vi "Dispatch Verify Queue.vi"(8 "error in (no error)":errorcluster, 9 "Timeout (100 ms)":i32=100, 10 "queue name":string, 11 "receiver host":string) -> (0 "error out":errorcluster, 2 "String Response":string, 3 "Message":T1)   [LabVIEW 2014, in "AMC.lvlib"]
uses:
  AMC.lvlib
  _SubVIs/Globals.vi
  Keyed Array/KeyedArray.ctl
  Keyed Array/Tools_KeyedArray.lvlib
  _SubVIs/TypeDefs/Message.ctl
panel:
  out "Response time (ms)":i32
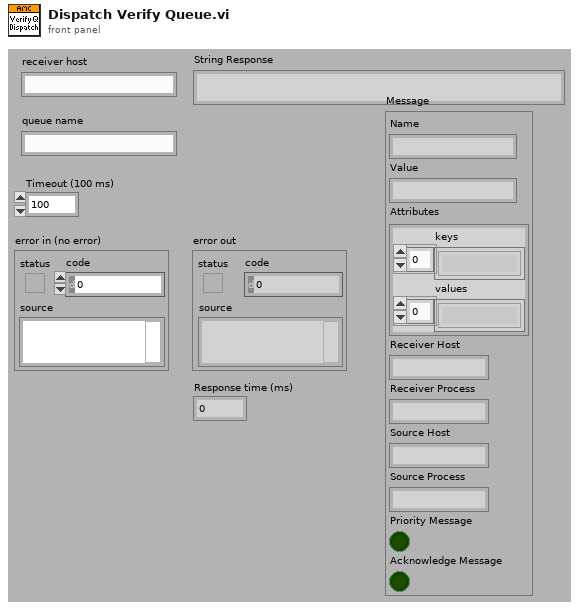
[diagram p1: front panel]
types:
  T1 = typedef "AMC.lvlib/Message.ctl" = cluster{"Name":string, "Value":string, "Attributes":T2, "Receiver Host":string, "Receiver Process":string, "Source Host":string, "Source Process":string, "Priority Message":bool, "Acknowledge Message":bool}
  T2 = typedef "Tools_KeyedArray.lvlib/KeyedArray.ctl" = cluster{"keys":string[], "values":string[]}
  T3 = typedef "AMC.lvlib/Message Queue.ctl" = refnum<queue>
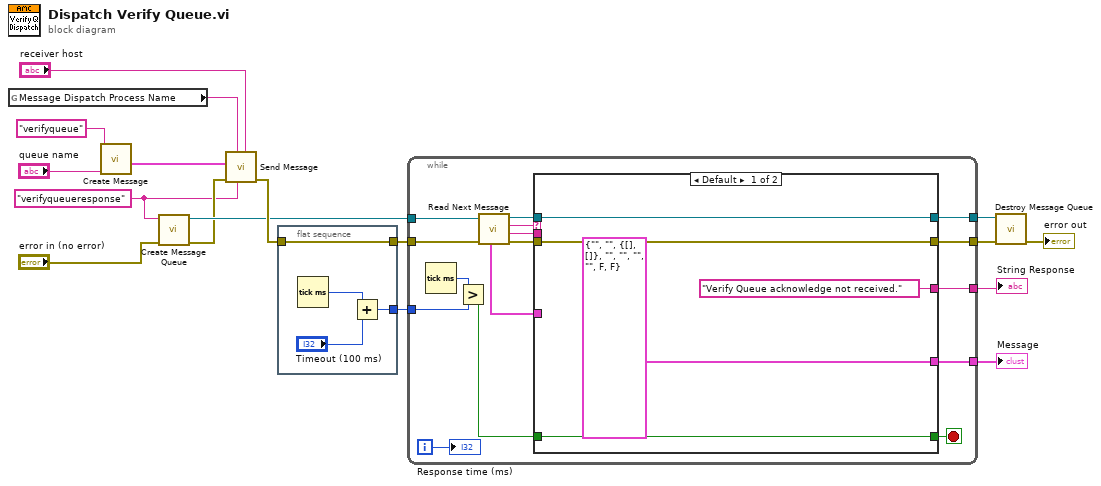
[diagram p0: block diagram]
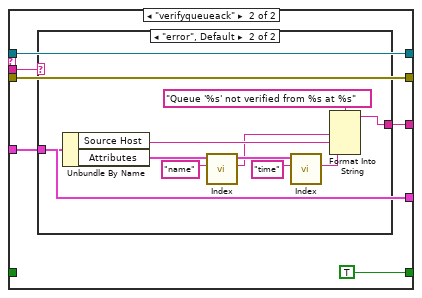
[diagram p2: hidden frame]
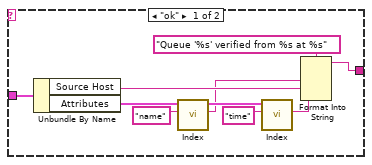
[diagram p3: hidden frame]
diagram:
  w3 = "verifyqueueresponse" ("message queue name")
  n1 = global read "Globals.vi" "Message Dispatch Process Name"() -> (w1:string)
  n2 = call "Create Message.vi"("Value"="queue name", "Name"="verifyqueue") -> ("Message"=w4:T1)  [unwired: 1 in, 8 out]
  n3 = call "Create Message Queue.vi"("error in (no error)"="error in (no error)", "Message Queue Name"=w3) -> ("error out"=w5:errorcluster, "Message Queue out"=w6:T3)  [unwired: 2 in, 6 out]
  n4 = call "Send Message.vi"("Receiver Host"="receiver host", "Source Process"=w3, "Receiver Process"=w1, "error in (no error)"=w5, "Message"=w4) -> ("error out"=w11:errorcluster)  [unwired: 3 in, 3 out]
  n5 = flat-sequence {
    tunnel: [w21] -> w10
    tunnel: w11 -> [w21]
    tunnel: [w18] -> w9
    frame #0 {
      n6 = Tick Count (ms)() -> (millisecond timer value=w20:u32)
      n7 = Add(x=w20, y="Timeout (100 ms)") -> (x+y=w18:u32)
    }
  }
  n8 = while {
    tunnel: w10 -> [w37]
    tunnel: [w34] -> w14
    tunnel: [w33] -> w13
    tunnel: [w30] -> w7
    tunnel: [w29] -> w8
    tunnel: w6 -> [w28]
    tunnel: w9 -> [w26]
    i -> [w23]
    stop <- w25 stop-if-true
    n9 = Tick Count (ms)() -> (millisecond timer value=w27:u32)
    n10 = Greater?(x=w27, y=w26) -> (0:w24:bool)
    n11 = call "Read Next Message.vi"("error in (no error)"=w37, "Message Queue in"=w28) -> ("error out"=w32:errorcluster, "Message Value"=w22:string, "Message Name"=w36:string, "Message Queue out"=w31:T3, "Message"=w35:T1)  [unwired: 3 in, 2 out]
    n12 = case shown="Default" w36 {
      tunnel: w35 -> [_ w47]
      tunnel: ["Verify Queue acknowledge not received." w48] -> w34
      tunnel: [T1 {"Name"="", "Value"="", "Attributes"={"keys"=[], "values"=[]}, "Receiver Host"="", "Receiver Process"="", "Source Host"="", "Source Process"="", "Priority Message"=FALSE, "Acknowledge Message"=FALSE} ("Message") w47] -> w33
      tunnel: [w39 w46] -> w30
      tunnel: w32 -> [w39 w46]
      tunnel: [w40 w45] -> w29
      tunnel: w31 -> [w40 w45]
      tunnel: [w38 TRUE] -> w25
      tunnel: w24 -> [w38 _]
      tunnel: w22 -> [_ w43]
      frame Default {
      }
      frame "verifyqueueack" {
        n13 = case shown="\"error\", Default" w43 {
          tunnel: [w54 w64] -> w48
          tunnel: w47 -> [w53 w63]
          frame "ok" {
            n14 = Unbundle By Name(w53) -> ("Source Host"=w58:string, "Attributes"=w51:T2)
            n15 = call "Index.vi"("key"="name", "array in"=w51) -> ("value"=w49:string, "duplicate array"=w50:T2)  [unwired: 2 in, 2 out]
            n16 = call "Index.vi"("key"="time", "array in"=w50) -> ("value"=w57:string)  [unwired: 2 in, 3 out]
            n17 = Format Into String(format string="Queue '%s' verified from %s at %s", w49, w58, w57) -> (resulting string=w54:string)  [unwired: 2 in, 1 out]
          }
          frame "error", Default {
            n18 = Unbundle By Name(w63) -> ("Source Host"=w68:string, "Attributes"=w61:T2)
            n19 = call "Index.vi"("key"="name", "array in"=w61) -> ("value"=w59:string, "duplicate array"=w60:T2)  [unwired: 2 in, 2 out]
            n20 = call "Index.vi"("key"="time", "array in"=w60) -> ("value"=w67:string)  [unwired: 2 in, 3 out]
            n21 = Format Into String(format string="Queue '%s' not verified from %s at %s", w59, w68, w67) -> (resulting string=w64:string)  [unwired: 2 in, 1 out]
          }
        }
      }
    }
    "Response time (ms)" <- w23
  }
  "String Response" <- w14
  "Message" <- w13
  n22 = call "Destroy Message Queue.vi"("error in (no error)"=w7, "Message Queue in"=w8) -> ("error out"=→"error out":errorcluster)  [unwired: 9 out]
